vi "ALTS Encode User Password for Authen version 2.vi"(11 "User Info":T1) -> (2 "User Value (encoded)":string, 3 "User Name":string)   [LabVIEW 2013]
uses:
  Controls/ALTS User Info.ctl
  Controls/ALTS User Group Enum2.ctl
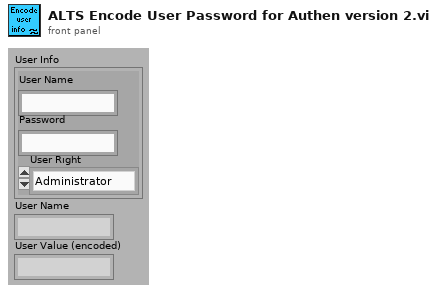
[diagram p1: front panel]
types:
  T1 = typedef "ALTS User Info.ctl" = cluster{"User Name":string, "Password":string, "User Right":T2}
  T2 = typedef "ALTS User Group Enum2.ctl" = enum16{"Administrator", "Super User", "Operator"}
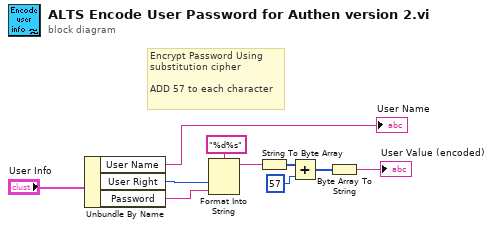
[diagram p0: block diagram]
diagram:
  # "Encrypt Password Using\nsubstitution cipher\n\nADD 57 to each character"
  n1 = Unbundle By Name("User Info") -> ("User Name"=→"User Name":string, "User Right"=w4:T2, "Password"=w3:string)
  n2 = Format Into String(format string="%d%s", w4, w3) -> (resulting string=w9:string)  [unwired: 2 in, 1 out]
  n3 = String To Byte Array(string=w9) -> (unsigned byte array=w6:u8[])
  n4 = Add(x=w6, y=57) -> (x+y=w7:i32[])
  n5 = Byte Array To String(unsigned byte array=w7) -> (string=→"User Value (encoded)":string)
